vi "intepret.vi"(8 "error in (no error)":errorcluster, 10 "context":string, 11 "OrExpression in":refnum<class "OrExpression.lvclass">) -> (0 "error out":errorcluster, 2 "result":bool, 3 "OrExpression out":refnum<class "OrExpression.lvclass">)   [LabVIEW 2018, in "OrExpression.lvclass"]
uses:
  OrExpression.lvclass
  OrExpression.lvclass/OrExpression.ctl
  TerminalExpression Class/TerminalExpression.lvclass
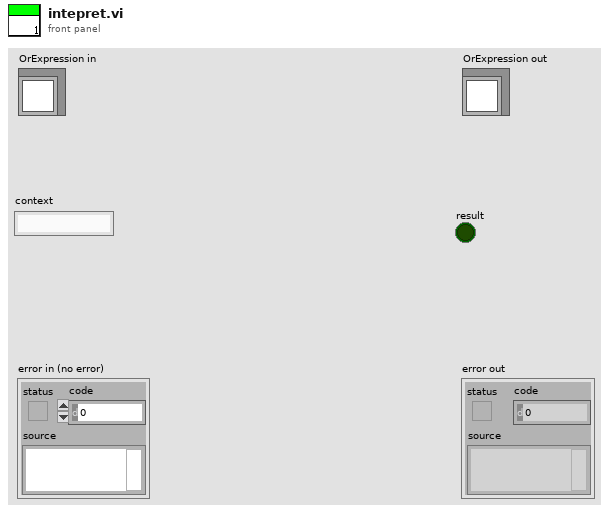
[diagram p1: front panel]
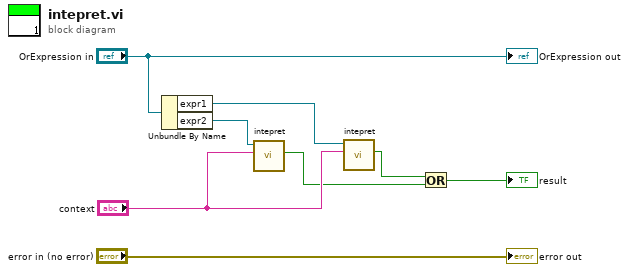
[diagram p0: block diagram]
diagram:
  n1 = Unbundle By Name("OrExpression in") -> ("expr1"=w5:refnum<class "TerminalExpression.lvclass">, "expr2"=w6:refnum<class "TerminalExpression.lvclass">)
  n2 = call-dynamic "intepret.vi"("context"="context", "TerminalExpression in"=w6) -> ("result"=w2:bool)  [unwired: 7 in, 2 out]
  n3 = call-dynamic "intepret.vi"("context"="context", "TerminalExpression in"=w5) -> ("result"=w3:bool)  [unwired: 7 in, 2 out]
  n4 = Or(x=w3, y=w2) -> (x .or. y?=→"result":bool)
  "error out" <- "error in (no error)"
  "OrExpression out" <- "OrExpression in"
